vi "HW_GEN - Parse PopUp Parameters from XML.vi"(10 "string in":string) -> (2 "PopUp":cluster{"Pop Type":T1, "string in":string})   [LabVIEW 2016]
uses:
  ToolKit/Popup/Private/Ctrls/POP_Data Type.ctl
panel:
  in  "Pop Type":T1
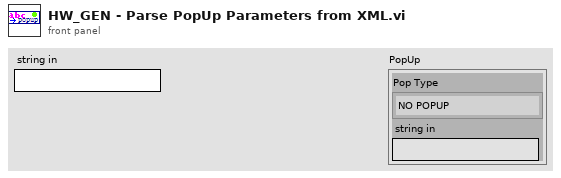
[diagram p1: front panel]
types:
  T1 = typedef "POP_Data Type.ctl" = enum16{"NO POPUP", "Unkown", "String", "Integer", "Float", "Color", "Boolean", "Ring", "Captioned String", "Captioned Integer", "Button Color", "2 Int Cluster", "4 Int Cluster", "6-Dbl Cluster", "Path", "Combox", "Time", "ShotCut String"}
  T2 = cluster{"index of element":i32, "string in":string}
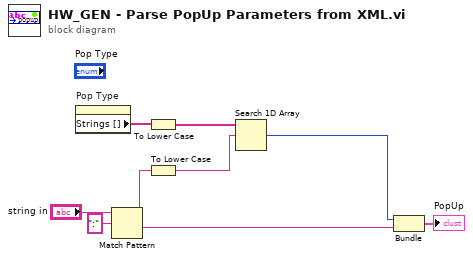
[diagram p0: block diagram]
diagram:
  n1 = property on="Pop Type" class="Enum (严格)"() -> ("Strings []"=w4:string[])  [unwired: 2 in, 2 out]
  n2 = Match Pattern(string="string in", regular expression=":" ("正则表达式")) -> (before substring=w7:string, after substring=w6:string)  [unwired: 1 in, 2 out]
  n3 = To Lower Case(string=w4) -> (all lower case string=w3:string[])
  n4 = To Lower Case(string=w7) -> (all lower case string=w2:string)
  n5 = Search 1D Array(1D array=w3, element=w2) -> (index of element=w1:i32)  [unwired: 1 in]
  n6 = Bundle("index of element"=w1, "string in"=w6) -> (→"PopUp":T2)  [unwired: 1 in]
